vi "setAcquisitionAbort.vi"(6 "Delay between send and receive [ms]":i32=100, 8 "error in (no error)":errorcluster, 10 "resetPort":i32, 11 "CCD in":refnum<class "CCD.lvclass">) -> (0 "error out":errorcluster, 1 "ID":i32, 2 "results-JSON string":string, 3 "CCD out":refnum<class "CCD.lvclass">)   [LabVIEW 2023, in "CCD.lvclass"]
uses:
  CCD.lvclass
  CCD.lvclass/CCD.ctl
  20f7d3bd-08ac-4524-9bed-df36c1da25a0.vi
  GenericDevice/GenericDevice.lvclass
  cab240a6-cbf4-4e2c-ab79-96d9c1b88265.vi
  <vilib>/IlluminatedG/lv-web-crypto/lv-json/JSON/JSON.lvlib
panel:
  # "Connector Pane"
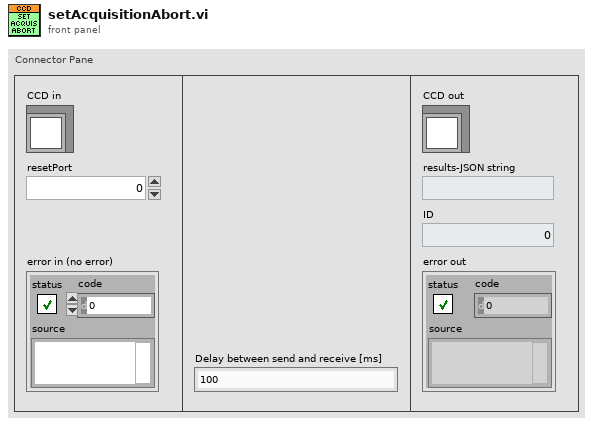
[diagram p1: front panel]
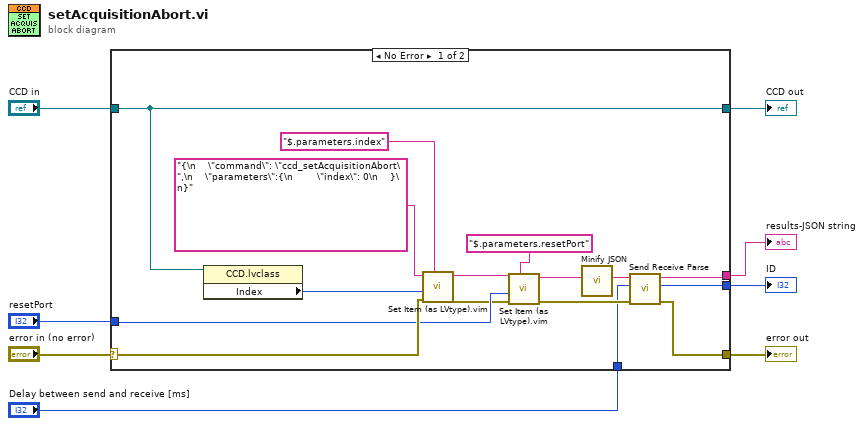
[diagram p0: block diagram]
diagram:
  n1 = case shown="No Error" "error in (no error)" {
    selector: "error in (no error)" -> [w20 w26]
    tunnel: [w14 w26] -> w7
    tunnel: [w22 w25] -> w5
    tunnel: "CCD in" -> [w22 w25]
    tunnel: "resetPort" -> [w18 _]
    tunnel: [w13 _] -> w4
    tunnel: [w12 _] -> w3
    tunnel: "Delay between send and receive [ms]" -> [w9 _]
    frame No Error {
      n2 = property class="CCD.lvclass"(reference=w22) -> ("Index"=w21:i32)  [unwired: 1 in, 2 out]
      n3 = call "Set Item (as LVtype).vim"("$Path or Item Name"="$.parameters.index", "error in (no error)"=w20, "Anything"=w21, "JSON"="{\n    \"command\": \"ccd_setAcquisitionAbort\",\n    \"parameters\":{\n        \"index\": 0\n    }\n}") -> ("error out"=w17:errorcluster, "<JSON>"=w15:string)  [unwired: 4 in, 1 out]
      n4 = call "Set Item (as LVtype).vim"("$Path or Item Name"="$.parameters.resetPort", "error in (no error)"=w17, "Anything"=w18, "JSON"=w15) -> ("error out"=w16:errorcluster, "<JSON>"=w11:string)  [unwired: 4 in, 1 out]
      n5 = call <vilib>:"Minify JSON.vi"("JSON String"=w11) -> ("Minified JSON"=w10:string)  [unwired: 10 in]
      n6 = call "Send Receive Parse.vi"("error in"=w16, "Delay between send and receive [ms]"=w9, "<JSON>"=w10) -> ("error out"=w14:errorcluster, "ID"=w12:i32, "results-JSON string"=w13:string)  [unwired: 6 in]
    }
    frame Error {
    }
  }
  "error out" <- w7
  "CCD out" <- w5
  "results-JSON string" <- w4
  "ID" <- w3
